vi "Hopper Control Telop.vi"(5 "Hopper Up/ Down Contol In":dbl, 6 "Hopper POT Initial Value":dbl) -> (0 "Hopper POT Calc Angle":dbl, 1 "Servo Angle":i32, 2 "Hopper Up/ Down Contol Out":dbl)   [LabVIEW 2016]
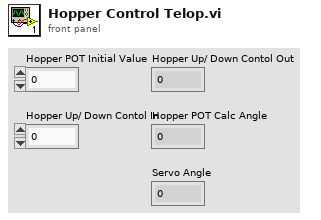
[diagram p1: front panel]
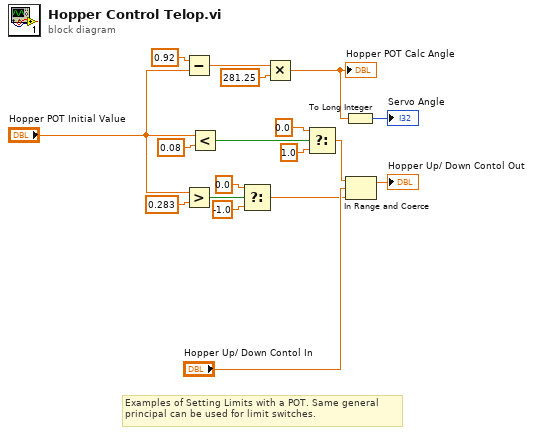
[diagram p0: block diagram]
diagram:
  # "Examples of Setting Limits with a POT. Same general\nprincipal can be used for limit switches."
  n1 = Subtract(x=0.92, y="Hopper POT Initial Value") -> (x-y=w12:dbl)
  n2 = Greater?(x="Hopper POT Initial Value", y=0.283) -> (0:w4:bool)
  n3 = Less?(x="Hopper POT Initial Value", y=0.08) -> (x < y?=w3:bool)
  n4 = Select(t=0.0, s=w4, f=-1.0) -> (s? t:f=w10:dbl)
  n5 = Multiply(x=w12, y=281.25) -> (x*y=w15:dbl)
  "Hopper POT Calc Angle" <- w15
  n6 = Select(t=0.0, s=w3, f=1.0) -> (s? t:f=w9:dbl)
  n7 = To Long Integer(number=w15) -> (32bit integer=→"Servo Angle":i32)
  n8 = In Range and Coerce(upper limit=w9, x="Hopper Up/ Down Contol In", lower limit=w10) -> (coerced(x)=→"Hopper Up/ Down Contol Out":dbl)  [unwired: 1 out]
